vi "NMR_Short_RF_Pulse_Sequence_V3.vi"() -> ()   [LabVIEW 2020]
uses:
  <instrlib>/niFgen/niFgen.llb/niFgen Waveform Type.ctl
  <instrlib>/niFgen/niFgen.llb/niFgen_ctl Trigger DigEdge - Edge Values (Ring).ctl
  <instrlib>/niFgen/niFgen.llb/niFgen_ctl Trigger Source Values (Ring).ctl
  <instrlib>/niFgen/niFgen.llb/niFgen Trigger Mode.ctl
  <instrlib>/niFgen/niFgen.llb/niFgen Output Mode.ctl
  <instrlib>/niFgen/niFgen.llb/niFgen Configure Digital Edge Start Trigger.vi
  <instrlib>/niFgen/niFgen.llb/niFgen Create Waveform (I16).vi
panel:
  in  "Sample Rate":dbl=50000000.0 format="%.2p"
  in  "Frequency":dbl=27500000.0 format="%.4p"
  in  "Delay Time (ms)":u32=4000
  in  "Number of Scans":i32=1
  in  "DC Offset":dbl(knob) scale=-0.5..0.5 scale format="%#.1f"
  in  "Gain":dbl(knob)=1.3 min=0.0 max=5.0 scale=0.0..5.0 scale format="%#.1f"
  in  "FGEN Resource Name 2":refnum<k15>="FGEN1" caption="FGEN Resource Name"
  in  "Waveform Information Array":T1(array[cluster])=[{"Waveform Type"=7, "Amplitude"=0.0, "# of points"=1000}, {"Waveform Type"=7, "Amplitude"=1.0, "# of points"=1200}, {"Waveform Type"=7, "Amplitude"=0.0, "# of points"=250000}, {"Waveform Type"=7, "Amplitude"=1.0, "# of points"=2400}, {"Waveform Type"=7, "Amplitude"=0.0, "# of points"=500000}, {"Waveform Type"=7, "Amplitude"=0.0, "# of points"=4000}, {"Waveform Type"=7, "Amplitude"=0.0, "# of points"=500000}, {"Waveform Type"=7, "Amplitude"=0.0, "# of points"=4000}, {"Waveform Type"=7, "Amplitude"=0.0, "# of points"=500000}, {"Waveform Type"=7, "Amplitude"=0.0, "# of points"=4000}, {"Waveform Type"=7, "Amplitude"=0.0, "# of points"=10000000}] {"Amplitude" min=0.0 max=1.0 format="%.2f"; "Waveform Type" items=["Sine", "Cosine", "Triangle", "Square", "Sawtooth", "Increasing Ramp", "Decreasing Ramp", "DC Value"]}
  in  "Amplitude":dbl=0.35 format="%0_3g"
  in  "FGEN Resource Name":refnum<k15>="Dev1"
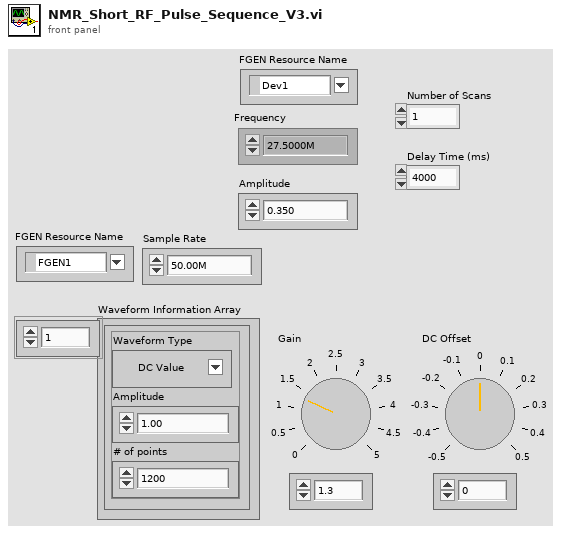
[diagram p1: front panel]
types:
  T1 = cluster{"Waveform Type":u16, "Amplitude":dbl, "# of points":u32}[]
  T2 = typedef "niFgen Output Mode.ctl" = u32
  T3 = typedef "niFgen Trigger Mode.ctl" = i32
  T4 = typedef "niFgen_ctl Trigger Source Values (Ring).ctl" = string
  T5 = typedef "niFgen_ctl Trigger DigEdge - Edge Values (Ring).ctl" = i32
  T6 = typedef "niFgen Waveform Type.ctl" = i32
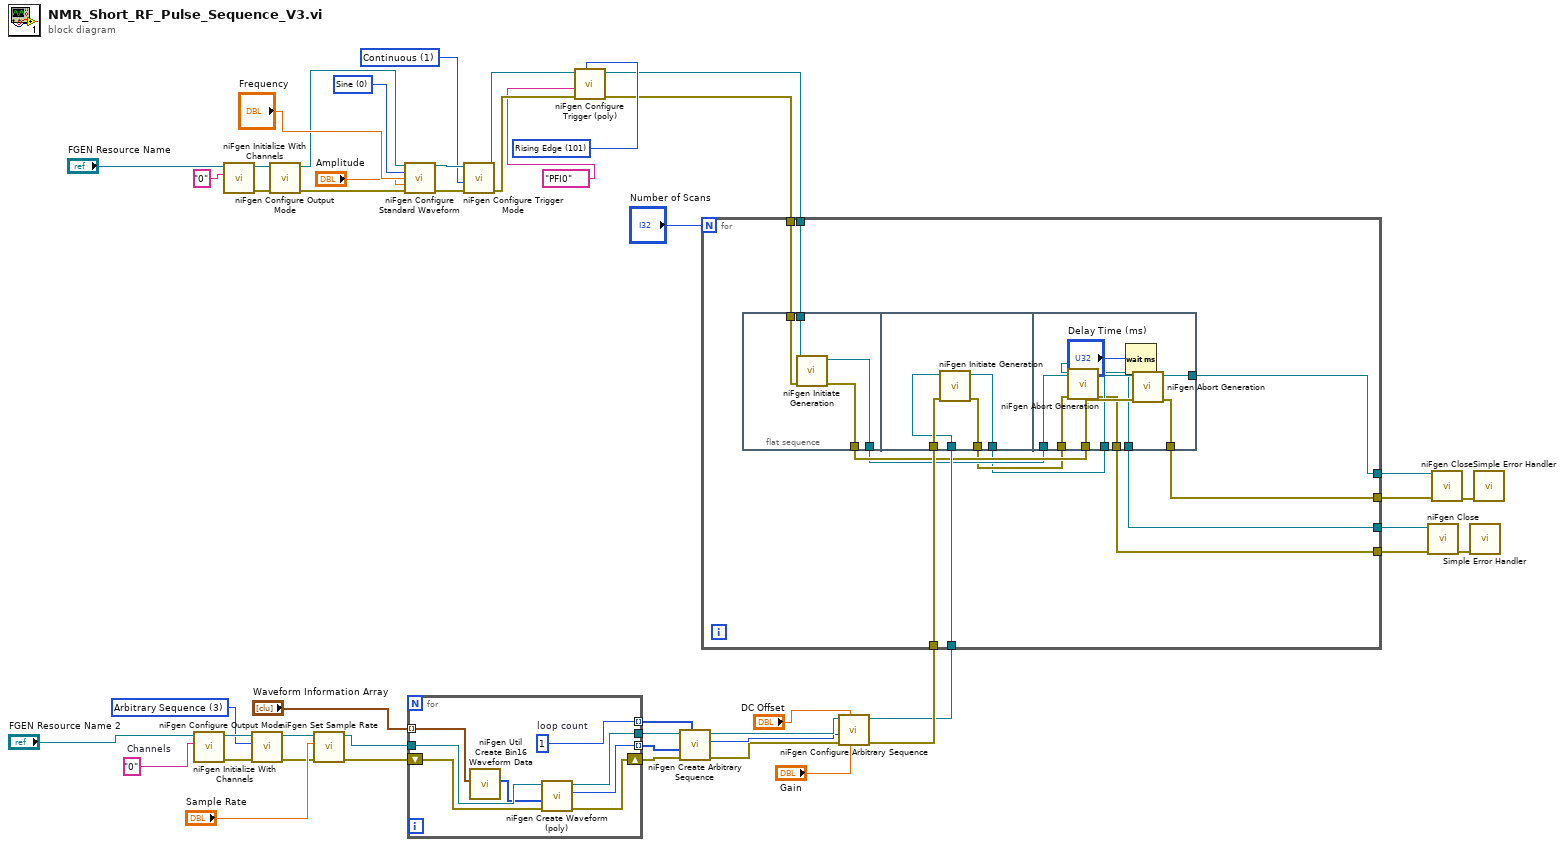
[diagram p0: block diagram]
diagram:
  w11 = "0"  # Channels
  w10 = T2 3 items=["Standard Function", "Frequency List", "Arbitrary Waveform", "Arbitrary Sequence", "Script"] ("output mode")
  w32 = T3 1 items=["Single", "Continuous", "Stepped", "Burst"] ("Trigger Mode (default: 1=continuous)")
  w35 = T5 101 items=["Rising Edge"=101, "Falling Edge"=102] ("Edge (Rising)")
  w33 = T6 0 items=["Sine", "Square", "Triangle", "Ramp Up", "Ramp Down", "DC", "Noise", "User"] ("Waveform")
  n1 = call <instrlib>:"niFgen Initialize With Channels.vi"("Channel Name"=w11, "Resource Name"="FGEN Resource Name 2") -> ("error out"=w21:errorcluster, "Instrument Handle Out"=w22:refnum<k15>)  [unwired: 8 in]
  n2 = call <instrlib>:"niFgen Initialize With Channels.vi"("Channel Name"="0", "Resource Name"="FGEN Resource Name") -> ("error out"=w39:errorcluster, "Instrument Handle Out"=w36:refnum<k15>)  [unwired: 8 in]
  n3 = call <instrlib>:"niFgen Configure Output Mode.vi"("error in (no error)"=w21, "Output Mode (default: 0=Standard Function)"=w10, "Instrument Handle"=w22) -> ("error out"=w27:errorcluster, "Instrument Handle Out"=w24:refnum<k15>)  [unwired: 6 in]
  n4 = call <instrlib>:"niFgen Configure Output Mode.vi"("error in (no error)"=w39, "Instrument Handle"=w36) -> ("error out"=w40:errorcluster, "Instrument Handle Out"=w37:refnum<k15>)  [unwired: 7 in]
  n5 = call <instrlib>:"niFgen Set Sample Rate.vi"("error in (no error)"=w27, "Sample Rate (Samp/s)"="Sample Rate", "Instrument Handle"=w24) -> ("error out"=w26:errorcluster, "Instrument Handle Out"=w25:refnum<k15>)  [unwired: 7 in]
  n6 = call <instrlib>:"niFgen Configure Standard Waveform.vi"("Instrument Handle"=w37, "Waveform"=w33, "Frequency"="Frequency", "Amplitude"="Amplitude", "error in (no error)"=w40) -> ("Instrument Handle Out"=w38:refnum<k15>, "error out"=w41:errorcluster)  [unwired: 9 in]
  n7 = for {
    shift-right: [w54] -> w17
    shift-left: w26 -> [w52]
    tunnel: [w55] -> w16
    tunnel: w25 -> [w53]
    tunnel: [w51] -> w15 mode=indexing
    tunnel: "Waveform Information Array" -> [w49] mode=indexing
    tunnel: [w48] -> w18 mode=indexing
    w48 = 1  # loop count
    n8 = call <instrlib>:"niFgen Util Create Bin16 Waveform Data.vi"("Waveform"=w49) -> ("Waveform Data"=w50:i16[])  [unwired: 10 in]
    n9 = call-poly <instrlib>:"niFgen Create Waveform (poly).vi"("error in (no error)"=w52, "Waveform Data Array"=w50, "Instrument Handle"=w53) -> ("error out"=w54:errorcluster, "Waveform Handle"=w51:i32, "Instrument Handle Out"=w55:refnum<k15>)  [unwired: 6 in]
  }
  n10 = call <instrlib>:"niFgen Configure Trigger Mode.vi"("error in (no error)"=w41, "Trigger Mode (default: 1=continuous)"=w32, "Instrument Handle"=w38) -> ("error out"=w45:errorcluster, "Instrument Handle Out"=w46:refnum<k15>)  [unwired: 7 in]
  n11 = call-poly <instrlib>:"niFgen Configure Trigger (poly).vi"("Edge (Rising)"=w35, "error in (no error)"=w45, "Source"=T4 "PFI0", "Instrument Handle"=w46) -> ("error out"=w30:errorcluster, "Instrument Handle Out"=w29:refnum<k15>)  [unwired: 6 in]
  n12 = call <instrlib>:"niFgen Create Arbitrary Sequence.vi"("Loop Counts Array"=w18, "error in (no error)"=w17, "Waveform Handles Array"=w15, "Instrument Handle"=w16) -> ("error out"=w12:errorcluster, "Sequence Handle"=w13:i32, "Instrument Handle Out"=w14:refnum<k15>)  [unwired: 5 in]
  n13 = call <instrlib>:"niFgen Configure Arbitrary Sequence.vi"("Gain"="Gain", "Offset"="DC Offset", "error in (no error)"=w12, "Sequence Handle"=w13, "Instrument Handle"=w14) -> ("error out"=w9:errorcluster, "Instrument Handle Out"=w8:refnum<k15>)  [unwired: 5 in]
  n14 = for {
    N: "Number of Scans" -> [_]
    tunnel: w30 -> [w67]
    tunnel: w29 -> [w66]
    tunnel: w9 -> [w65]
    tunnel: w8 -> [w64]
    tunnel: [w61] -> w5
    tunnel: [w60] -> w4
    tunnel: [w57] -> w2
    tunnel: [w56] -> w1
    n15 = flat-sequence {
      tunnel: [w71] -> w62
      tunnel: [w70] -> w63
      tunnel: w67 -> [w69]
      tunnel: w66 -> [w68]
      tunnel: [w75] -> w59
      tunnel: [w74] -> w58
      tunnel: w65 -> [w73]
      tunnel: w64 -> [w72]
      tunnel: w63 -> [w84]
      tunnel: w62 -> [w83]
      tunnel: [w82] -> w61
      tunnel: [w81] -> w60
      tunnel: w59 -> [w80]
      tunnel: w58 -> [w79]
      tunnel: [w78] -> w57
      tunnel: [w77] -> w56
      frame #0 {
        n16 = call <instrlib>:"niFgen Initiate Generation.vi"("error in (no error)"=w69, "Instrument Handle"=w68) -> ("error out"=w70:errorcluster, "Instrument Handle Out"=w71:refnum<k15>)  [unwired: 8 in]
      }
      frame #1 {
        n17 = call <instrlib>:"niFgen Initiate Generation.vi"("error in (no error)"=w73, "Instrument Handle"=w72) -> ("error out"=w75:errorcluster, "Instrument Handle Out"=w74:refnum<k15>)  [unwired: 8 in]
      }
      frame #2 {
        n18 = call <instrlib>:"niFgen Abort Generation.vi"("error in (no error)"=w80, "Instrument Handle"=w79) -> ("error out"=w78:errorcluster, "Instrument Handle Out"=w77:refnum<k15>)  [unwired: 8 in]
        n19 = Wait (ms)(milliseconds to wait="Delay Time (ms)") -> ()  [unwired: 1 out]
        n20 = call <instrlib>:"niFgen Abort Generation.vi"("error in (no error)"=w84, "Instrument Handle"=w83) -> ("error out"=w82:errorcluster, "Instrument Handle Out"=w81:refnum<k15>)  [unwired: 8 in]
      }
    }
  }
  n21 = call <instrlib>:"niFgen Close.vi"("error in (no error)"=w2, "Instrument Handle"=w1) -> ("error out"=w3:errorcluster)  [unwired: 9 in]
  n22 = call <instrlib>:"niFgen Close.vi"("error in (no error)"=w5, "Instrument Handle"=w4) -> ("error out"=w6:errorcluster)  [unwired: 9 in]
  n23 = call <vilib>:"Simple Error Handler.vi"("error in (no error)"=w3) -> ()  [unwired: 4 in, 5 out]
  n24 = call <vilib>:"Simple Error Handler.vi"("error in (no error)"=w6) -> ()  [unwired: 4 in, 5 out]
